vi "AverageColors.vi"(2 "ColorData":dbl, 3 "CurrentArray":dbl[](array[numeric])) -> (0 "UpdatedArray":dbl[](array[numeric]), 1 "Average":dbl)   [LabVIEW 2012]
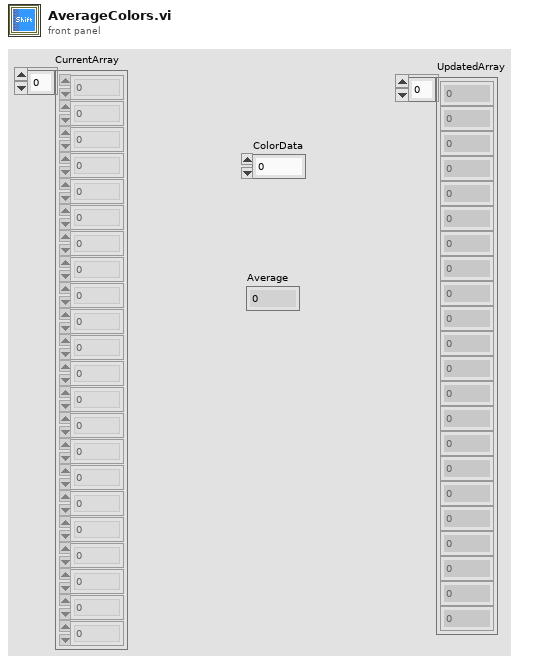
[diagram p1: front panel]
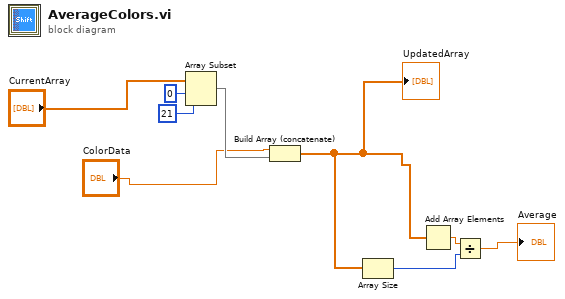
[diagram p0: block diagram]
diagram:
  n1 = Array Subset(array="CurrentArray", index=0, length=21) -> (w6:dbl[])
  n2 = Build Array (concatenate)("ColorData", w6) -> (w2:dbl[])
  "UpdatedArray" <- w2
  n3 = Array Size(array=w2) -> (size(s)=w1:i32)
  n4 = Add Array Elements(numeric array=w2) -> (sum=w4:dbl)
  n5 = Divide(x=w4, y=w1) -> (x/y=→"Average":dbl)
